vi "DigitalOscilloscope.vi"() -> ()   [LabVIEW 2014]
panel:
  in  "stop":bool
  out "error out":errorcluster
  out "Waveform Graph":dynamicdata(graph)
  in  "Cluster":T1
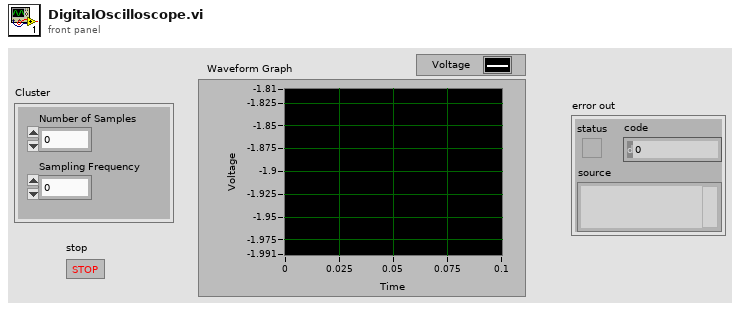
[diagram p1: front panel]
types:
  T1 = cluster{"Number of Samples":dbl, "Sampling Frequency":dbl}
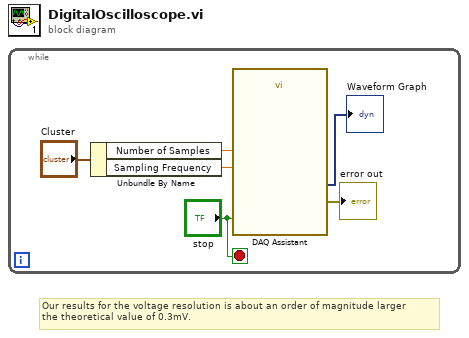
[diagram p0: block diagram]
diagram:
  # "Our results for the voltage resolution is about an order of magnitude larger \nthe theoretical value of 0.3mV."
  n1 = while {
    stop <- "stop" stop-if-true
    n2 = Unbundle By Name("Cluster") -> ("Number of Samples"=w5:dbl, "Sampling Frequency"=w4:dbl)
    n3 = call "DAQ Assistant"("rate"=w4, "number of samples"=w5, "stop (T)"="stop") -> ("data"=→"Waveform Graph":dynamicdata, "error out"=→"error out":errorcluster)  [unwired: 14 in, 1 out]
  }
